vi "Historicos.vi"() -> ()   [LabVIEW 2018]
uses:
  <vilib>/RAFA Solutions/Harmony UI Controls Kit/String & Path/String Indicator.ctl
  <vilib>/RAFA Solutions/Harmony UI Controls Kit/Boolean/OK Button.ctl
  <vilib>/RAFA Solutions/Harmony UI Controls Kit/Boolean/Blank Button - Green.ctl
  Controls/Hora y Fecha control.ctl
  Global/globalEventos.vi
  <vilib>/addons/database/Connection.llb/DB Tools Open Connec (Path).vi
  <vilib>/RAFA Solutions/Harmony UI Controls Kit/Flat UI Design.lvlib
  <vilib>/addons/database/NI_Database_API.lvlib
panel:
  in  "Nombre del Equipo":u16(ring) items=["EQUIPO_1", "EQUIPO_2", "EQUIPO_3", "EQUIPO_4", "EQUIPO_5", "EQUIPO_6"]
  out "fecha y hora":T1
  out "Historico":cluster{dbl[], dbl[]}[](graph)
  in  "exportar a excel":T2
  in  "Tiempo Final":timestamp format="%<%X\n%x>T"
  in  "Tiempo Inicio":timestamp format="%<%X\n%x>T"
  in  "Consultar":T2
  out "Generador":string
  in  "volver":T3
  out "Eventos":T4
  # "Sistema de Monitoreo de Calidad de Energía"
  # "Límites de tolerancia según IEEE45"
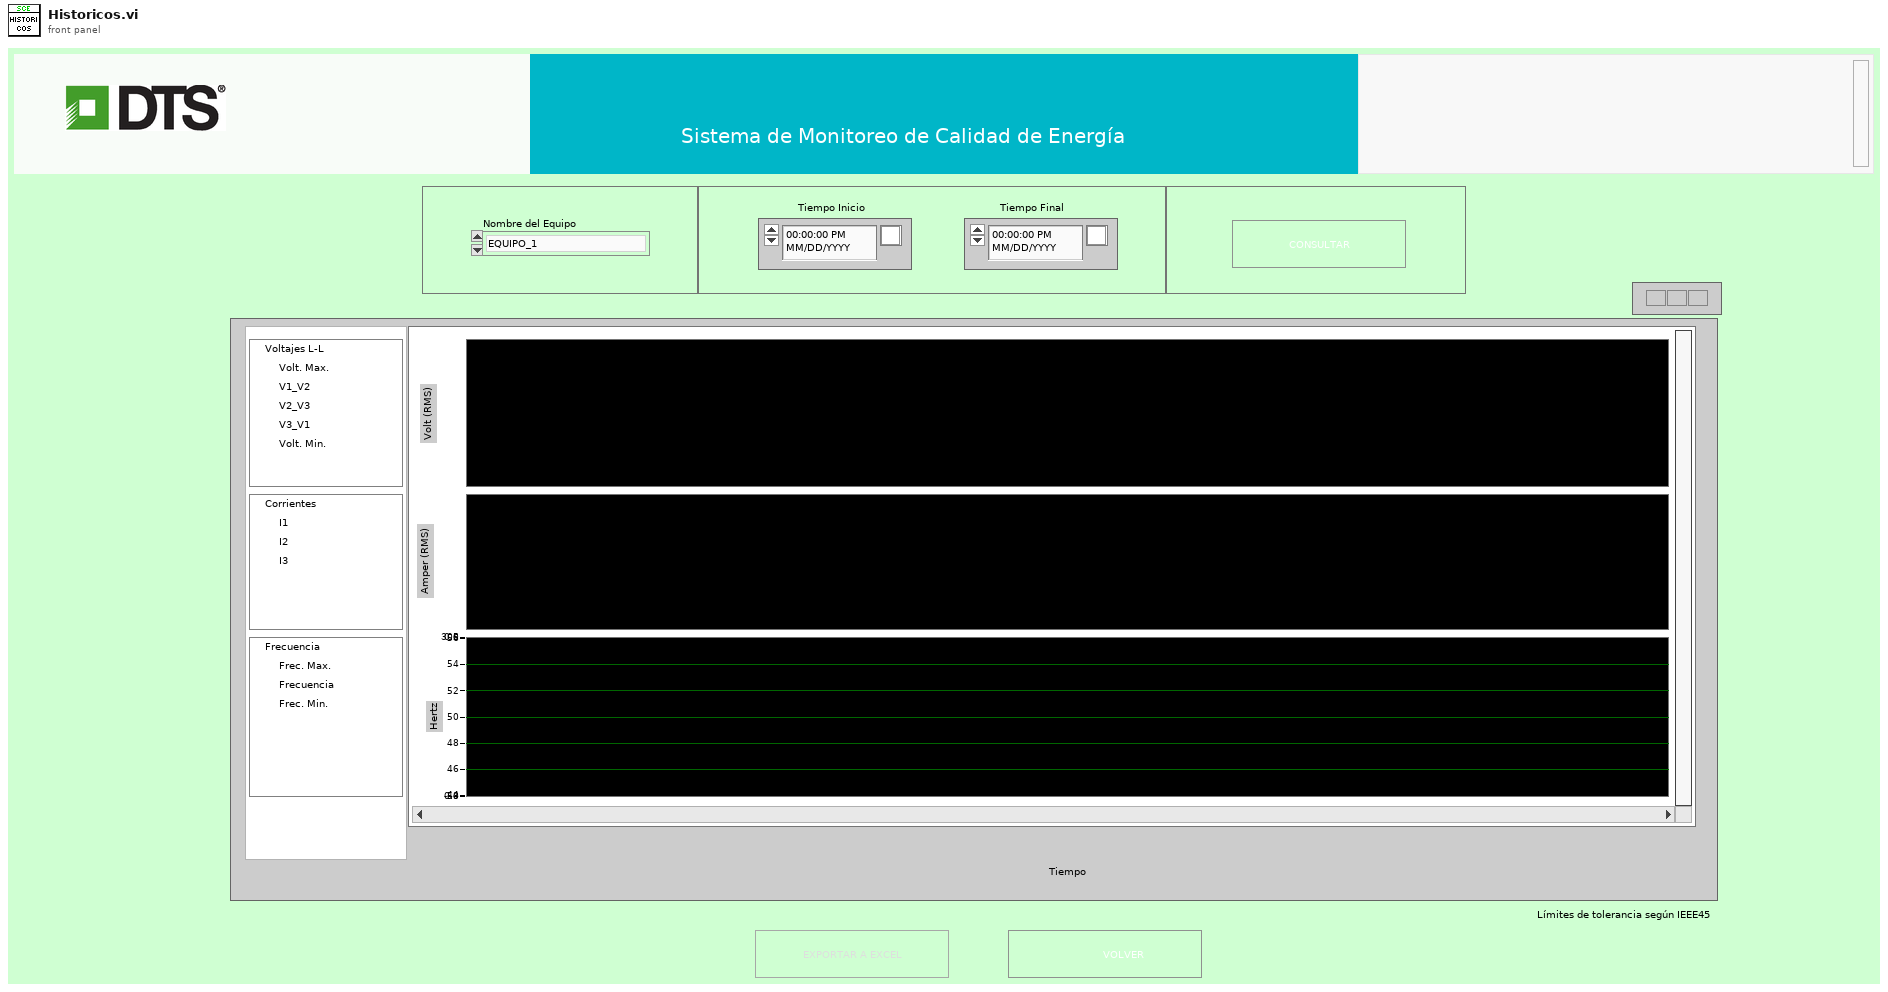
[diagram p1: front panel]
types:
  T1 = typedef "Hora y Fecha control.ctl" = cluster{"fecha":string, "dia semana":string, "fecha 2":string}
  T2 = typedef "Flat UI Design.lvlib/Blank Button - Green.ctl" = bool
  T3 = typedef "Flat UI Design.lvlib/OK Button.ctl" = bool
  T4 = typedef "Flat UI Design.lvlib/String Indicator.ctl" = string
  T5 = typedef "NI_Database_API.lvlib/Conn ObjectReference.ctl" = refnum<k1>
  T6 = enum8{"Enabled", "Disabled", "Disabled and Grayed Out"}
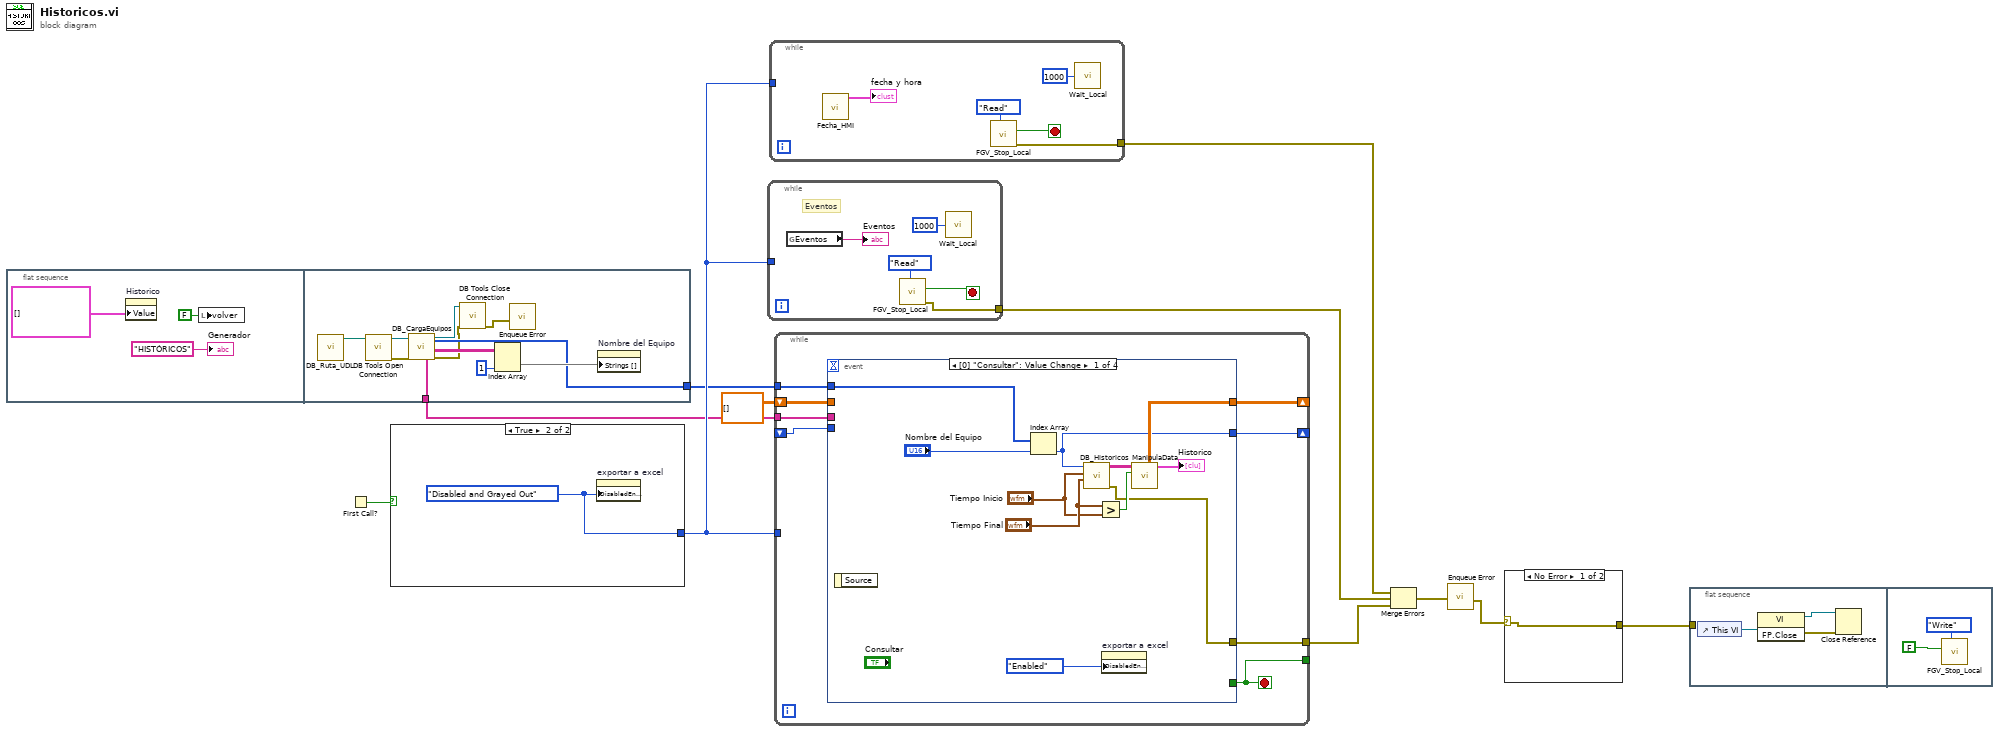
[diagram p0: block diagram]
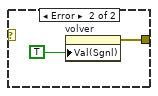
[diagram p2: hidden frame]
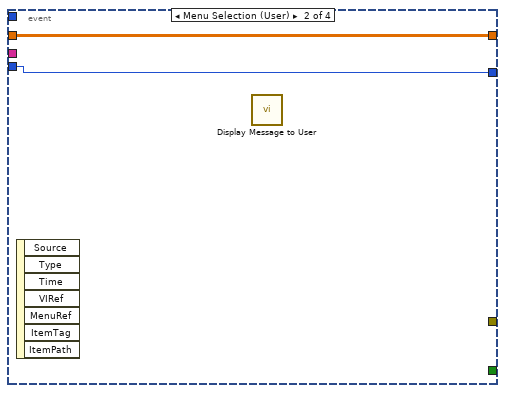
[diagram p4: hidden frame]
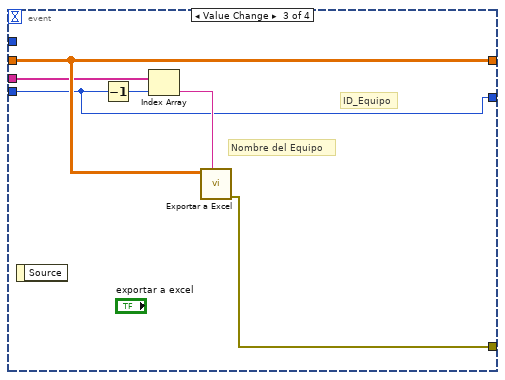
[diagram p5: hidden frame]
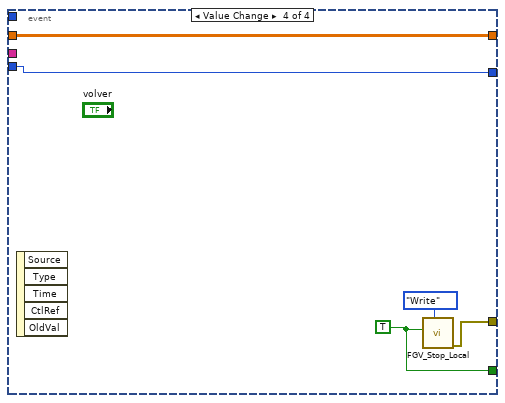
[diagram p6: hidden frame]
diagram:
  n1 = flat-sequence {
    tunnel: [w19] -> w7
    tunnel: [w15] -> w3
    frame #0 {
      n2 = property on="Historico" class="MixedGraph (strict)"("Value"=cluster{dbl[], dbl[]}[] [] ("Historico")) -> ()  [unwired: 2 in, 2 out]
      n3 = local write "volver"(T3 FALSE ("volver")) -> ()
      "Generador" <- "HISTÓRICOS" ("Generador in")
    }
    frame #1 {
      n4 = call "DB_Ruta_UDL.vi"() -> ("UDL ruta"=w24:path)  [unwired: 11 in]
      n5 = call-poly <vilib>:"DB Tools Open Connection.vi"("connection information"=w24) -> ("error out"=w18:errorcluster, "connection reference"=w23:T5)  [unwired: 7 in]
      n6 = call "DB_CargaEquipos.vi"("error in (no error)"=w18, "db in"=w23) -> ("error out"=w17:errorcluster, "Equipos"=w21:string[][], "db out"=w22:T5, "NOMBRE_EQUIPOS"=w15:string[], "ID_EQUIPOS"=w19:i32[])  [unwired: 2 in, 3 out]
      n7 = call <vilib>:"DB Tools Close Connection.vi"("error in (no error)"=w17, "connection reference"=w22) -> ("error out"=w16:errorcluster)  [unwired: 5 in]
      n8 = Index Array(array=w21, index (col)=1 ("disabled index (col)")) -> (element=w25:string[])  [unwired: 1 in]
      n9 = call "Enqueue Error.vi"("error in"=w16) -> ()  [unwired: 9 in, 2 out]
      n10 = property on="Nombre del Equipo" class="Ring (strict)"("Strings []"=w25) -> ()  [unwired: 2 in, 2 out]
    }
  }
  n11 = First Call?() -> (First Call?: T/F=w11:bool)
  n12 = case shown="True" w11 {
    tunnel: [_ w26] -> w10
    frame False {
    }
    frame True {
      w26 = T6."Disabled and Grayed Out" ("Disabled")
      n13 = property on="exportar a excel" class="Bool"("DisabledEnum"=w26) -> ()  [unwired: 2 in, 2 out]
    }
  }
  n14 = while {
    tunnel: w10 -> [_]
    tunnel: [w27] -> w1
    stop <- w30 stop-if-true
    # "Eventos"
    n15 = global read "globalEventos.vi" "Eventos"() -> (→"Eventos":string)
    n16 = call "FGV_Stop_Local.vi"("Action"=enum16{"Read", "Write"}."Read") -> ("Error Out"=w27:errorcluster, "Var Out"=w30:bool)  [unwired: 9 in]
    n17 = call "Wait_Local.vi"("Wait time (msec)"=u32 1000 ("milliseconds to wait")) -> ()  [unwired: 5 in]
  }
  n18 = while {
    tunnel: w10 -> [_]
    tunnel: [w33] -> w9
    stop <- w34 stop-if-true
    n19 = call "Fecha_HMI.vi"() -> ("fecha y hora"=→"fecha y hora":T1)  [unwired: 11 in]
    n20 = call "FGV_Stop_Local.vi"("Action"=enum16{"Read", "Write"}."Read") -> ("Error Out"=w33:errorcluster, "Var Out"=w34:bool)  [unwired: 9 in]
    n21 = call "Wait_Local.vi"("Wait time (msec)"=u32 1000 ("milliseconds to wait")) -> ()  [unwired: 5 in]
  }
  n22 = while {
    shift-right: [w44] -> _
    shift-left: dbl[][] [] ("Data a exportar") -> [w43]
    tunnel: w10 -> [_]
    tunnel: [w42] -> _
    tunnel: [w41] -> w8
    tunnel: w7 -> [w40]
    shift-right: [w39] -> _
    shift-left: _ -> [w37]
    tunnel: w3 -> [w38]
    stop <- w42 stop-if-true
    n23 = event shown="[0] \"Consultar\": Value Change" {
      selector: _ -> [_ _ _ _]
      dyn-events: _ -> [_ _ _ _]
      timeout: _ -> [_ _ _ _]
      tunnel: [w54 w57 w63 w65] -> w44
      tunnel: w43 -> [_ w57 w63 w65]
      tunnel: [_ _ _ w67] -> w42
      tunnel: [w46 _ w62 w66] -> w41
      tunnel: w40 -> [w48 _ _ _]
      tunnel: [w45 w56 w59 w64] -> w39
      tunnel: w38 -> [_ _ w61 _]
      tunnel: w37 -> [_ w56 w59 w64]
      event Value Change {
        n24 = event-data() -> ()  [unwired: 1 in, 1 out]
        n25 = Index Array(array=w48, index="Nombre del Equipo") -> (element=w45:i32)
        n26 = call "DB_Historicos.vi"("Final"="Tiempo Final", "Inicio"="Tiempo Inicio", "ID_EQUIPO"=w45) -> ("error out"=w46:errorcluster, "Data"=w55:string[][])  [unwired: 7 in]
        n27 = Greater?(x="Tiempo Final", y="Tiempo Inicio") -> (0:w49:bool)
        n28 = property on="exportar a excel" class="Bool"("DisabledEnum"=T6."Enabled" ("Disabled")) -> ()  [unwired: 2 in, 2 out]
        n29 = call "ManipulaData.vi"("Error en fechas?"=w49, "Data In"=w55) -> ("Historico Out"=→"Historico":cluster{dbl[], dbl[]}[], "Data a exportar"=w54:dbl[][])  [unwired: 8 in]
      }
      event Menu Selection (User) {
        n30 = event-data() -> ()  [unwired: 1 in, 7 out]
        n31 = call "Display Message to User"() -> ()  [unwired: 10 in, 2 out]
      }
      event Value Change {
        # "ID_Equipo"
        # "Nombre del Equipo"
        n32 = event-data() -> ()  [unwired: 1 in, 1 out]
        n33 = Decrement(x=w59) -> (x-1=w58:i32)
        n34 = Index Array(array=w61, index=w58) -> (element=w60:string)
        n35 = call "Exportar a Excel.vi"("Nombre Equipo"=w60, "Data"=w63) -> ("error out"=w62:errorcluster)  [unwired: 9 in]
      }
      event Value Change {
        w67 = TRUE
        n36 = event-data() -> ()  [unwired: 1 in, 5 out]
        n37 = call "FGV_Stop_Local.vi"("Action"=enum16{"Read", "Write"}."Write", "Var In"=w67) -> ("Error Out"=w66:errorcluster)  [unwired: 8 in, 1 out]
      }
    }
  }
  n38 = Merge Errors(w9, w1, w8) -> (w6:errorcluster)
  n39 = call "Enqueue Error.vi"("error in"=w6) -> ("error out"=w5:errorcluster)  [unwired: 9 in, 1 out]
  n40 = case shown="No Error" w5 {
    selector: w5 -> [w69 _]
    tunnel: [w69 w70] -> w4
    frame No Error {
    }
    frame Error {
      n41 = property on="volver" class="Bool (strict)"("Val(Sgnl)"=TRUE) -> (error out=w70:errorcluster)  [unwired: 2 in, 1 out]
    }
  }
  n42 = flat-sequence {
    tunnel: w4 -> [_]
    frame #0 {
      n43 = control-ref of="This VI"() -> (w74:refnum<vi>)
      n44 = invoke class="VI" method="FP.Close"(reference=w74) -> (reference out=w73:refnum<vi>, error out=w72:errorcluster)  [unwired: 2 in, 1 out]
      n45 = Close Reference(reference=w73, error in (no error)=w72) -> ()  [unwired: 1 out]
    }
    frame #1 {
      n46 = call "FGV_Stop_Local.vi"("Action"=enum16{"Read", "Write"}."Write", "Var In"=FALSE) -> ()  [unwired: 8 in, 2 out]
    }
  }
